vi "Periodic TasksXX.vi"(8 "error in":errorcluster) -> ()   [LabVIEW 2019]
doc: "This VI runs in parallel to other tasks. It can contain as many user-defined periodic loops as you need. These can carry out PID or other sorts of timed response."
uses:
  <vilib>/Rock Robotics/WPI/Utilities/WPI_GetSetVariantRefNum.vi
  Robot Global Data.vi
  <vilib>/addons/control/pid/pid.llb/PID (DBL).vi
  <vilib>/Rock Robotics/Network Tables/NT Write Numeric Array.vi
  <vilib>/Rock Robotics/Network Tables/NT Write Number.vi
  <vilib>/Rock Robotics/Network Tables/NT Write Boolean.vi
  Secret_Control_Library_Protected/Secret_Control_Library_Protected.lvlib
  <vilib>/addons/control/pid/NI_PID_pid.lvlib
  <vilib>/Rock Robotics/WPI/ThirdParty/JAS_Junk/TrajLib/Trajectory_Library.lvlib
panel:
  in  "Speed PID":T1={"proportional gain (Kc)"=0.6, "integral time (Ti, min)"=0.015, "derivative time (Td, min)"=0.0} {"derivative time (Td, min)" format="%.3f"; "integral time (Ti, min)" format="%.3f"; "proportional gain (Kc)" format="%.3f"}
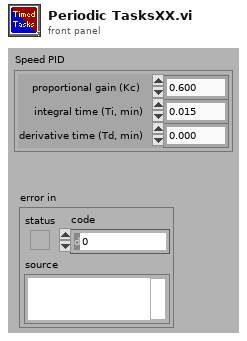
[diagram p1: front panel]
types:
  T1 = cluster{"proportional gain (Kc)":dbl, "integral time (Ti, min)":dbl, "derivative time (Td, min)":dbl}
  T2 = typedef "WPI_EncoderDevRef.ctl" = cluster{"DevStatus":errorcluster, "EncoderIndex":T3, "CounterIndex":T4, "DistancePerCount":dbl, "Decoding Type":T5}
  T3 = typedef "FPGA_EncoderIdx.ctl" = enum8{"Enc 0", "Enc 1", "Enc 2", "Enc 3", "Enc 4", "Enc 5", "Enc 6", "Enc 7", "Invalid"}
  T4 = typedef "FPGA_CounterCtrSystemIndex.ctl" = enum8{"Ctr 0", "Ctr 1", "Ctr 2", "Ctr 3", "Ctr 4", "Ctr 5", "Ctr 6", "Ctr 7", "Invalid"}
  T5 = typedef "WPI_EncoderType.ctl" = enum16{"1x", "2x", "4x"}
  T6 = typedef "WPI_GyroDevRef.ctl" = cluster{"DevStatus":errorcluster, "Analog Channel":T7, "Gain (VoltsPerDegree/Second)":dbl, "Gyro Type":enum16{"Analog", "XRS450"}, "Handle":i32, "SPI Bus":T8, "Device Found":bool, "Sample Rate":dbl, "Calibrate On Open":bool, "Offset":dbl}
  T7 = typedef "FPGA_AIChannel.ctl" = enum8{"AI 0", "AI 1", "AI 2", "AI 3", "AI MXP 0", "AI MXP 1", "AI MXP 2", "AI MXP 3", "Invalid"}
  T8 = typedef "spi_bus.ctl" = enum16{"SPI On-Board, CS0", "SPI On-Board, CS1", "SPI On-Board, CS2", "SPI On-Board, CS3", "SPI MXP", "Invalid"}
  T9 = typedef "WPI_RobotDriveDevRef.ctl" = cluster{"DevStatus":errorcluster, "Motors[]":T10[], "Square Inputs":bool, "Max Output":dbl}
  T10 = typedef "WPI_MotorControlDeviceRef.ctl" = cluster{"DeviceStatus":errorcluster, "Type":T11, "PWM":cluster{"PWM Channel":T12, "DeadBand":T13}, "CAN":cluster{"Device Number":u8, "SetOutput VI Ref":variant, "GetOutput VI Ref":variant, "Enable VI Ref":variant, "Disable VI Ref":variant, "Data":variant}, "Invert":bool, "DIO PWM":cluster{"PWM \"Enable\" Channel":T12, "DIOChannel":T14, "PWM Rate":dbl}}
  T11 = typedef "WPI_MotorControlType.ctl" = enum16{"PWM", "CAN", "DIO PWM"}
  T12 = typedef "FPGA_DIOPWMChannel.ctl" = enum8{"PWM 0", "PWM 1", "PWM 2", "PWM 3", "PWM 4", "PWM 5", "PWM 6", "PWM 7", "PWM 8", "PWM 9", "PWM MXP 0", "PWM MXP 1", "PWM MXP 2", "PWM MXP 3", "PWM MXP 4", "PWM MXP 5", "PWM MXP 6", "PWM MXP 7", "PWM MXP 8", "PWM MXP 9", "Invalid"}
  T13 = typedef "WPI_PWMDeadband.ctl" = cluster{"Name":string, "maxPositivePwm":i32, "minPositivePwm":i32, "centerPwm":i32, "maxNegativePwm":i32, "minNegativePwm":i32, "angularRange":u16}
  T14 = typedef "FPGA_DIOChannel.ctl" = enum8{"DIO 0", "DIO 1", "DIO 2", "DIO 3", "DIO 4", "DIO 5", "DIO 6", "DIO 7", "DIO 8", "DIO 9", "DIO MXP 0", "DIO MXP 1", "DIO MXP 2", "DIO MXP 3", "DIO MXP 4", "DIO MXP 5", "DIO MXP 6", "DIO MXP 7", "DIO MXP 8", "DIO MXP 9", "DIO MXP 10", "DIO MXP 11", "DIO MXP 12", "DIO MXP 13", "DIO MXP 14", "DIO MXP 15", "SPI Port CS1", "SPI Port CS2", "SPI Port CS3", "SPI Port MISO", "SPI Port MOSI", "Invalid"}
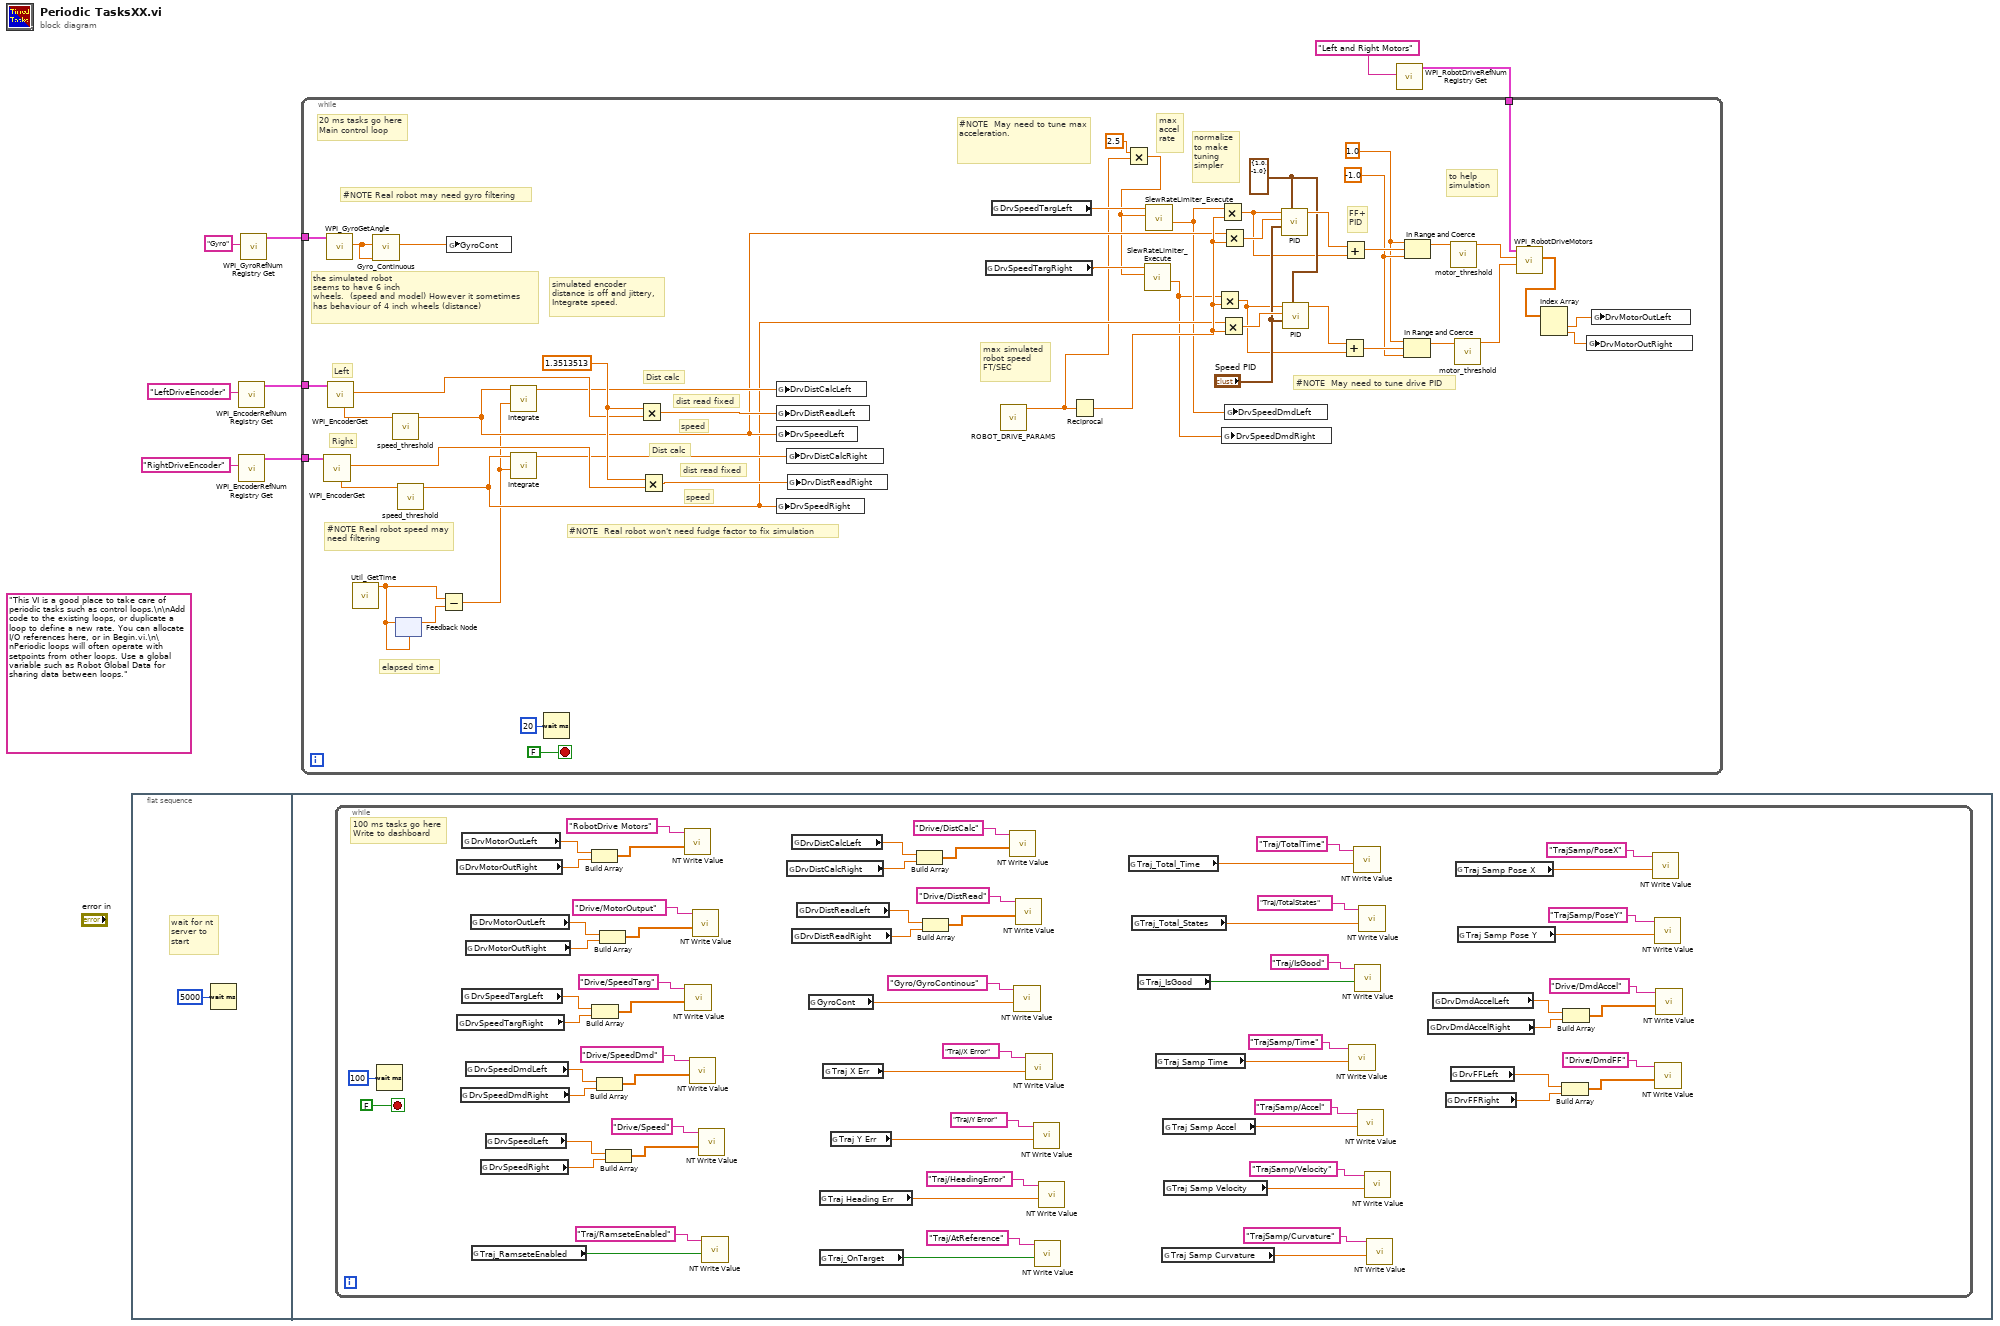
[diagram p0: block diagram]
diagram:
  (unwired) "This VI is a good place to take care of periodic tasks such as control loops.\n\nAdd code to the existing loops, or duplicate a loop to define a new rate. You can allocate I/O references here, or in Begin.vi.\n\nPeriodic loops will often operate with setpoints from other loops. Use a global variable such as Robot Global Data for sharing data between loops."
  n1 = flat-sequence {
    frame #0 {
      # "wait for nt\nserver to \nstart"
      n2 = Wait (ms)(milliseconds to wait=u32 5000) -> ()  [unwired: 1 out]
    }
    frame #1 {
      n3 = while {
        stop <- FALSE stop-if-true
        # "100 ms tasks go here\nWrite to dashboard"
        n4 = Wait (ms)(milliseconds to wait=u32 100) -> ()  [unwired: 1 out]
        n5 = global read "Robot Global Data.vi" "DrvMotorOutRight"() -> (w74:dbl)
        n6 = global read "Robot Global Data.vi" "DrvSpeedTargRight"() -> (w66:dbl)
        n7 = global read "Robot Global Data.vi" "DrvSpeedDmdRight"() -> (w62:dbl)
        n8 = global read "Robot Global Data.vi" "DrvMotorOutLeft"() -> (w75:dbl)
        n9 = global read "Robot Global Data.vi" "DrvSpeedTargLeft"() -> (w67:dbl)
        n10 = global read "Robot Global Data.vi" "DrvMotorOutRight"() -> (w70:dbl)
        n11 = global read "Robot Global Data.vi" "DrvSpeedDmdLeft"() -> (w63:dbl)
        n12 = global read "Robot Global Data.vi" "DrvMotorOutLeft"() -> (w71:dbl)
        n13 = global read "Robot Global Data.vi" "Traj_RamseteEnabled"() -> (w10:bool)
        n14 = global read "Robot Global Data.vi" "DrvSpeedRight"() -> (w58:dbl)
        n15 = global read "Robot Global Data.vi" "DrvSpeedLeft"() -> (w59:dbl)
        n16 = Build Array(w75, w74) -> (w73:dbl[])
        n17 = Build Array(w67, w66) -> (w65:dbl[])
        n18 = Build Array(w63, w62) -> (w61:dbl[])
        n19 = Build Array(w71, w70) -> (w69:dbl[])
        n20 = Build Array(w59, w58) -> (w57:dbl[])
        n21 = call-poly <vilib>:"NT Write Value.vi"("Numeric Array"=w73, "Name"="RobotDrive Motors") -> ()  [unwired: 9 in, 1 out]
        n22 = call-poly <vilib>:"NT Write Value.vi"("Numeric Array"=w65, "Name"="Drive/SpeedTarg") -> ()  [unwired: 9 in, 1 out]
        n23 = call-poly <vilib>:"NT Write Value.vi"("Numeric Array"=w61, "Name"="Drive/SpeedDmd") -> ()  [unwired: 9 in, 1 out]
        n24 = call-poly <vilib>:"NT Write Value.vi"("Numeric Array"=w69, "Name"="Drive/MotorOutput") -> ()  [unwired: 9 in, 1 out]
        n25 = call-poly <vilib>:"NT Write Value.vi"("Numeric Array"=w57, "Name"="Drive/Speed") -> ()  [unwired: 9 in, 1 out]
        n26 = call-poly <vilib>:"NT Write Value.vi"("Boolean"=w10, "Name"="Traj/RamseteEnabled") -> ()  [unwired: 9 in, 1 out]
        n27 = global read "Robot Global Data.vi" "DrvDistCalcRight"() -> (w54:dbl)
        n28 = global read "Robot Global Data.vi" "DrvDistCalcLeft"() -> (w55:dbl)
        n29 = global read "Robot Global Data.vi" "DrvDistReadRight"() -> (w50:dbl)
        n30 = global read "Robot Global Data.vi" "DrvDistReadLeft"() -> (w51:dbl)
        n31 = global read "Robot Global Data.vi" "GyroCont"() -> (w46:dbl)
        n32 = global read "Robot Global Data.vi" "Traj Heading Err"() -> (w40:dbl)
        n33 = global read "Robot Global Data.vi" "Traj_OnTarget"() -> (w38:bool)
        n34 = global read "Robot Global Data.vi" "Traj X Err"() -> (w44:dbl)
        n35 = global read "Robot Global Data.vi" "Traj Y Err"() -> (w42:dbl)
        n36 = Build Array(w55, w54) -> (w53:dbl[])
        n37 = Build Array(w51, w50) -> (w49:dbl[])
        n38 = call-poly <vilib>:"NT Write Value.vi"("Numeric Array"=w53, "Name"="Drive/DistCalc") -> ()  [unwired: 9 in, 1 out]
        n39 = call-poly <vilib>:"NT Write Value.vi"("Numeric"=w46, "Name"="Gyro/GyroContinous") -> ()  [unwired: 9 in, 1 out]
        n40 = call-poly <vilib>:"NT Write Value.vi"("Numeric Array"=w49, "Name"="Drive/DistRead") -> ()  [unwired: 9 in, 1 out]
        n41 = call-poly <vilib>:"NT Write Value.vi"("Numeric"=w44, "Name"="Traj/X Error") -> ()  [unwired: 9 in, 1 out]
        n42 = call-poly <vilib>:"NT Write Value.vi"("Numeric"=w42, "Name"="Traj/Y Error") -> ()  [unwired: 9 in, 1 out]
        n43 = call-poly <vilib>:"NT Write Value.vi"("Boolean"=w38, "Name"="Traj/AtReference") -> ()  [unwired: 9 in, 1 out]
        n44 = call-poly <vilib>:"NT Write Value.vi"("Numeric"=w40, "Name"="Traj/HeadingError") -> ()  [unwired: 9 in, 1 out]
        n45 = global read "Robot Global Data.vi" "Traj_Total_Time"() -> (w34:dbl)
        n46 = global read "Robot Global Data.vi" "Traj_Total_States"() -> (w33:dbl)
        n47 = global read "Robot Global Data.vi" "Traj_IsGood"() -> (w32:bool)
        n48 = global read "Robot Global Data.vi" "Traj Samp Time"() -> (w28:dbl)
        n49 = global read "Robot Global Data.vi" "Traj Samp Curvature"() -> (w31:dbl)
        n50 = global read "Robot Global Data.vi" "Traj Samp Accel"() -> (w29:dbl)
        n51 = global read "Robot Global Data.vi" "Traj Samp Velocity"() -> (w30:dbl)
        n52 = call-poly <vilib>:"NT Write Value.vi"("Numeric"=w28, "Name"="TrajSamp/Time") -> ()  [unwired: 9 in, 1 out]
        n53 = call-poly <vilib>:"NT Write Value.vi"("Numeric"=w34, "Name"="Traj/TotalTime") -> ()  [unwired: 9 in, 1 out]
        n54 = call-poly <vilib>:"NT Write Value.vi"("Boolean"=w32, "Name"="Traj/IsGood") -> ()  [unwired: 9 in, 1 out]
        n55 = call-poly <vilib>:"NT Write Value.vi"("Numeric"=w29, "Name"="TrajSamp/Accel") -> ()  [unwired: 9 in, 1 out]
        n56 = call-poly <vilib>:"NT Write Value.vi"("Numeric"=w33, "Name"="Traj/TotalStates") -> ()  [unwired: 9 in, 1 out]
        n57 = call-poly <vilib>:"NT Write Value.vi"("Numeric"=w30, "Name"="TrajSamp/Velocity") -> ()  [unwired: 9 in, 1 out]
        n58 = call-poly <vilib>:"NT Write Value.vi"("Numeric"=w31, "Name"="TrajSamp/Curvature") -> ()  [unwired: 9 in, 1 out]
        n59 = global read "Robot Global Data.vi" "DrvDmdAccelRight"() -> (w19:dbl)
        n60 = global read "Robot Global Data.vi" "DrvDmdAccelLeft"() -> (w18:dbl)
        n61 = global read "Robot Global Data.vi" "DrvFFRight"() -> (w22:dbl)
        n62 = global read "Robot Global Data.vi" "DrvFFLeft"() -> (w21:dbl)
        n63 = global read "Robot Global Data.vi" "Traj Samp Pose X"() -> (w16:dbl)
        n64 = global read "Robot Global Data.vi" "Traj Samp Pose Y"() -> (w17:dbl)
        n65 = Build Array(w21, w22) -> (w23:dbl[])
        n66 = Build Array(w18, w19) -> (w20:dbl[])
        n67 = call-poly <vilib>:"NT Write Value.vi"("Numeric"=w16, "Name"="TrajSamp/PoseX") -> ()  [unwired: 9 in, 1 out]
        n68 = call-poly <vilib>:"NT Write Value.vi"("Numeric"=w17, "Name"="TrajSamp/PoseY") -> ()  [unwired: 9 in, 1 out]
        n69 = call-poly <vilib>:"NT Write Value.vi"("Numeric Array"=w23, "Name"="Drive/DmdFF") -> ()  [unwired: 9 in, 1 out]
        n70 = call-poly <vilib>:"NT Write Value.vi"("Numeric Array"=w20, "Name"="Drive/DmdAccel") -> ()  [unwired: 9 in, 1 out]
      }
    }
  }
  n71 = call <vilib>:"WPI_EncoderRefNum Registry Get.vi"("refnum name"="LeftDriveEncoder") -> ("EncoderDevRef"=w6:T2)  [unwired: 9 in, 1 out]
  n72 = call <vilib>:"WPI_EncoderRefNum Registry Get.vi"("refnum name"="RightDriveEncoder") -> ("EncoderDevRef"=w7:T2)  [unwired: 9 in, 1 out]
  n73 = call <vilib>:"WPI_GyroRefNum Registry Get.vi"("refnum name"="Gyro") -> ("GyroDevRef"=w2:T6)  [unwired: 9 in, 1 out]
  n74 = call <vilib>:"WPI_RobotDriveRefNum Registry Get.vi"("refnum name"="Left and Right Motors") -> ("RobotDriveDevRef"=w1:T9)  [unwired: 1 in, 9 out]
  n75 = while {
    tunnel: w7 -> [w121]
    tunnel: w6 -> [w120]
    tunnel: w2 -> [w118]
    tunnel: w1 -> [w104]
    stop <- FALSE stop-if-true
    w113 = -1.0 ("lower limit")
    w112 = 1.0 ("upper limit")
    w110 = cluster{"output high":dbl, "output low":dbl} {"output high"=1.0, "output low"=-1.0} ("output range")
    w124 = 1.3513513
    # "#NOTE  Real robot won't need fudge factor to fix simulation"
    # "#NOTE  May need to tune drive PID"
    # "#NOTE  May need to tune max acceleration."
    # "elapsed time"
    # "to help\nsimulation"
    # "#NOTE Real robot speed may need filtering"
    # "max simulated\nrobot speed\nFT/SEC"
    # "max\naccel\nrate"
    # "normalize\nto make\ntuning\nsimpler"
    # "FF+\nPID"
    # "#NOTE Real robot may need gyro filtering"
    # "Right"
    # "Left"
    # "the simulated robot\nseems to have 6 inch\nwheels.  (speed and model) However it sometimes\nhas behaviour of 4 inch wheels (distance)"
    # "speed"
    # "dist read fixed"
    # "Dist calc"
    # "speed"
    # "dist read fixed"
    # "Dist calc"
    # "simulated encoder\ndistance is off and jittery,\nIntegrate speed."
    # "20 ms tasks go here\nMain control loop"
    n76 = call <vilib>:"WPI_EncoderGet.vi"("EncoderDevRef"=w121) -> ("Distance"=w122:dbl, "Rate"=w93:dbl)  [unwired: 5 in, 4 out]
    n77 = call <vilib>:"WPI_GyroGetAngle.vi"("GyroDevRef"=w118) -> ("Angle"=w119:dbl)  [unwired: 7 in, 3 out]
    n78 = call <vilib>:"WPI_EncoderGet.vi"("EncoderDevRef"=w120) -> ("Distance"=w123:dbl, "Rate"=w95:dbl)  [unwired: 5 in, 4 out]
    n79 = call <vilib>:"Util_GetTime.vi"() -> ("FPGA_Time_Seconds"=w85:dbl)  [unwired: 10 in, 1 out]
    n80 = call "Gyro_Continuous.vi"("GyroInitial"=w119, "GyroInput"=w119) -> ("GyroContinuous"=w87:dbl)  [unwired: 9 in]
    n81 = call "speed_threshold.vi"("SPEED IN"=w95) -> ("SPEED OUT"=w94:dbl)  [unwired: 10 in]
    n82 = feedback-in #1(w85) -> ()
    n83 = feedback #1(w85) -> (w86:dbl)
    n84 = call "speed_threshold.vi"("SPEED IN"=w93) -> ("SPEED OUT"=w92:dbl)  [unwired: 10 in]
    n85 = Subtract(x=w85, y=w86) -> (x-y=w84:dbl)
    n86 = global write "Robot Global Data.vi" "GyroCont"(w87) -> ()
    n87 = call "Integrate.vi"("Elapsed Sec"=w84, "Rate"=w94) -> ("DIST"=w103:dbl)  [unwired: 9 in]
    n88 = call "Integrate.vi"("Elapsed Sec"=w84, "Rate"=w92) -> ("DIST"=w101:dbl)  [unwired: 9 in]
    n89 = Wait (ms)(milliseconds to wait=u32 20) -> ()  [unwired: 1 out]
    n90 = Multiply(x=w124, y=w123) -> (x*y=w102:dbl)
    n91 = Multiply(x=w124, y=w122) -> (x*y=w100:dbl)
    n92 = global write "Robot Global Data.vi" "DrvDistCalcLeft"(w103) -> ()
    n93 = global write "Robot Global Data.vi" "DrvDistReadLeft"(w102) -> ()
    n94 = global write "Robot Global Data.vi" "DrvSpeedLeft"(w94) -> ()
    n95 = global write "Robot Global Data.vi" "DrvSpeedRight"(w92) -> ()
    n96 = global write "Robot Global Data.vi" "DrvDistCalcRight"(w101) -> ()
    n97 = global write "Robot Global Data.vi" "DrvDistReadRight"(w100) -> ()
    n98 = global read "Robot Global Data.vi" "DrvSpeedTargRight"() -> (w80:dbl)
    n99 = global read "Robot Global Data.vi" "DrvSpeedTargLeft"() -> (w82:dbl)
    n100 = call "ROBOT_DRIVE_PARAMS.vi"() -> ("Max Speed Ft/Sec"=w78:dbl)  [unwired: 10 in, 1 out]
    n101 = Reciprocal(x=w78) -> (1/x=w96:dbl)
    n102 = Multiply(x=2.5, y=w78) -> (x*y=w79:dbl)
    n103 = call <vilib>:"SlewRateLimiter_Execute.vi"("Rate"=w79, "Input"=w80) -> ("Output"=w81:dbl)  [unwired: 8 in, 1 out]
    n104 = call <vilib>:"SlewRateLimiter_Execute.vi"("Rate"=w79, "Input"=w82) -> ("Output"=w83:dbl)  [unwired: 8 in, 1 out]
    n105 = Multiply(x=w81, y=w96) -> (x*y=w107:dbl)
    n106 = Multiply(x=w83, y=w96) -> (x*y=w106:dbl)
    n107 = Multiply(x=w92, y=w96) -> (x*y=w111:dbl)
    n108 = Multiply(x=w94, y=w96) -> (x*y=w108:dbl)
    n109 = global write "Robot Global Data.vi" "DrvSpeedDmdRight"(w81) -> ()
    n110 = global write "Robot Global Data.vi" "DrvSpeedDmdLeft"(w83) -> ()
    n111 = call-poly <vilib>:"PID.vi"("output range"=w110, "PID gains"="Speed PID", "process variable"=w108, "setpoint"=w106) -> ("output"=w117:dbl)  [unwired: 6 in, 1 out]
    n112 = call-poly <vilib>:"PID.vi"("output range"=w110, "PID gains"="Speed PID", "process variable"=w111, "setpoint"=w107) -> ("output"=w115:dbl)  [unwired: 6 in, 1 out]
    n113 = Add(x=w115, y=w107) -> (x+y=w114:dbl)
    n114 = Add(x=w117, y=w106) -> (x+y=w116:dbl)
    n115 = In Range and Coerce(upper limit=w112, x=w114, lower limit=w113) -> (coerced(x)=w89:dbl)  [unwired: 1 out]
    n116 = In Range and Coerce(upper limit=w112, x=w116, lower limit=w113) -> (coerced(x)=w90:dbl)  [unwired: 1 out]
    n117 = call "motor_threshold.vi"("motor in"=w90) -> ("motor out"=w91:dbl)  [unwired: 10 in]
    n118 = call "motor_threshold.vi"("motor in"=w89) -> ("motor out"=w88:dbl)  [unwired: 10 in]
    n119 = call <vilib>:"WPI_RobotDriveMotors.vi"("RightSpeed"=w88, "LeftSpeed"=w91, "RobotDriveDevRef"=w104) -> ("Motor Values"=w99:dbl[])  [unwired: 6 in, 2 out]
    n120 = Index Array(array=w99) -> (element #1=w98:dbl, element #2=w97:dbl)  [unwired: 2 in]
    n121 = global write "Robot Global Data.vi" "DrvMotorOutRight"(w97) -> ()
    n122 = global write "Robot Global Data.vi" "DrvMotorOutLeft"(w98) -> ()
  }
